vi "Menu_Case Selector Terminal.vi"(11 "Affected Items":T1) -> (3 "Menu Items To Add":T2(array[cluster]))   [LabVIEW 2023]
uses:
  top/BundleMagic.ctl
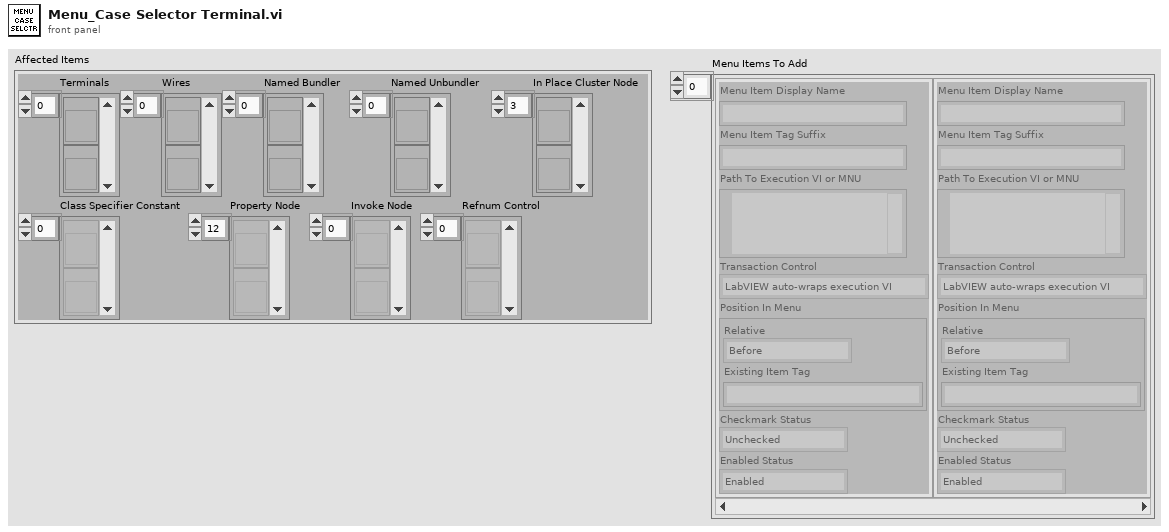
[diagram p1: front panel]
types:
  T1 = typedef "BundleMagic.ctl" = cluster{"Terminals":refnum<vi>[], "Wires":refnum<vi>[], "Named Bundler":refnum<vi>[], "Named Unbundler":refnum<vi>[], "In Place Cluster Node":refnum<vi>[], "Class Specifier Constant":refnum<vi>[], "Property Node":refnum<vi>[], "Invoke Node":refnum<vi>[], "Refnum Control":refnum<vi>[]}
  T2 = cluster{"Menu Item Display Name":string, "Menu Item Tag Suffix":string, "Path To Execution VI or MNU":path, "Transaction Control":enum8{"LabVIEW auto-wraps execution VI", "Execution VI will define if needed"}, "Position In Menu":cluster{"Relative":enum8{"Before", "Instead of", "After", "Into Submenu"}, "Existing Item Tag":string}, "Checkmark Status":enum8{"Unchecked", "Checked"}, "Enabled Status":enum8{"Enabled", "Disabled"}}[]
  T3 = cluster{"Relative":enum8{"Before", "Instead of", "After", "Into Submenu"}, "Existing Item Tag":string}
  T4 = enum16{"[NONE]", "Wire Bundle", "Wire Unbundle", "Terminal Unbundle", "Terminal Bundle", "Bundler Insert", "Bundler Remove", "Bundler Remove Unwired", "Bundler Rearrange", "In Place Insert", "In Place Remove", "In Place Remove Unwired", "In Place Rearrange", "Wire Properties", "Wire Method", "Terminal Properties", "Terminal Method", "Properties Insert", "Properties Remove", "Properties Remove Unwired", "Properties Rearrange", "Method Change", "Class for Constant", "Class For Control", "Class For Node", "Class Name to Clipboard"}[]
  T5 = cluster{"Relative":enum8{"Before", "Instead of", "After", "Into Submenu"}, "Existing Item Tag":string}[]
  T6 = cluster{"Menu Item Display Name":string, "Menu Item Tag Suffix":string, "Path To Execution VI or MNU":path, "Transaction Control":enum8{"LabVIEW auto-wraps execution VI", "Execution VI will define if needed"}, "Position In Menu":cluster{"Relative":enum8{"Before", "Instead of", "After", "Into Submenu"}, "Existing Item Tag":string}, "Checkmark Status":enum8{"Unchecked", "Checked"}, "Enabled Status":enum8{"Enabled", "Disabled"}}
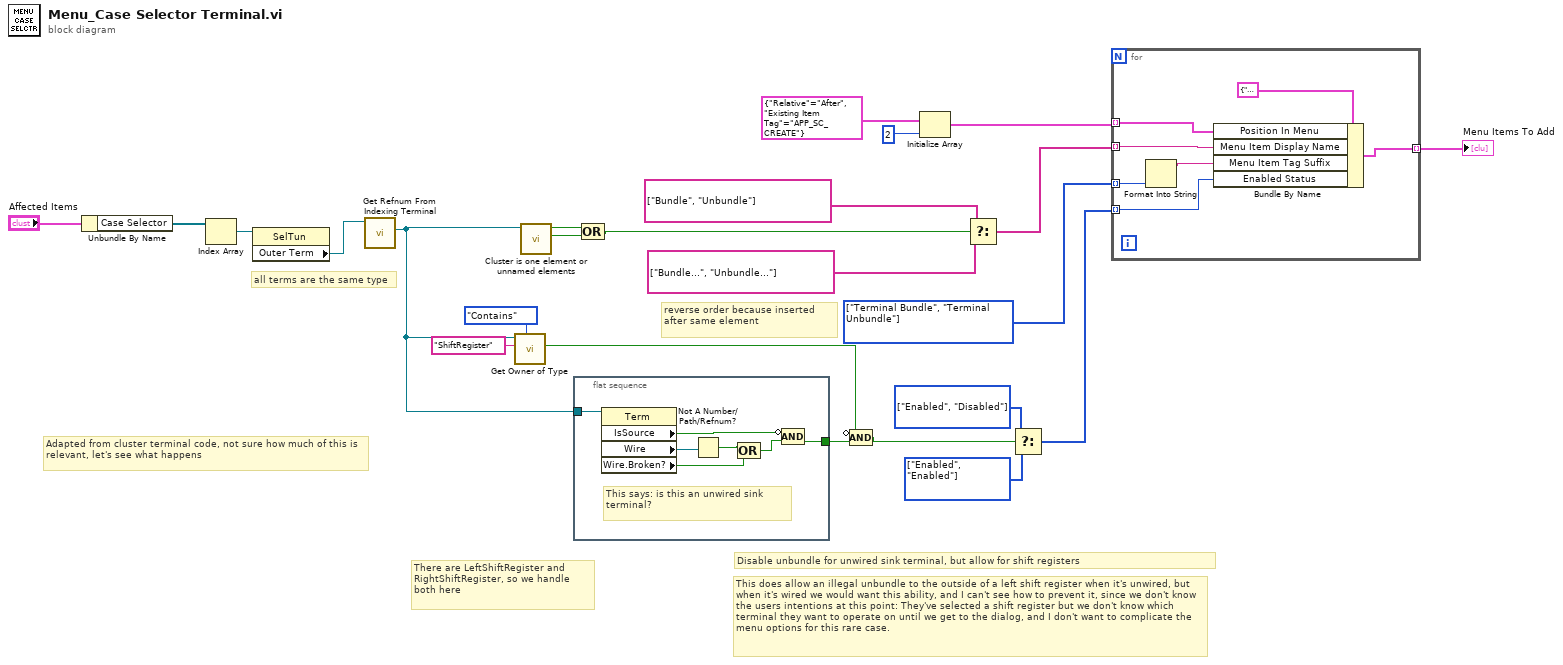
[diagram p0: block diagram]
diagram:
  w13 = T4 [enum."Terminal Bundle", enum."Terminal Unbundle"] items=["[NONE]", "Wire Bundle", "Wire Unbundle", "Terminal Unbundle", "Terminal Bundle", "Bundler Insert", "Bundler Remove", "Bundler Remove Unwired", "Bundler Rearrange", "In Place Insert", "In Place Remove", "In Place Remove Unwired", "In Place Rearrange", "Wire Properties", "Wire Method", "Terminal Properties", "Terminal Method", "Properties Insert", "Properties Remove", "Properties Remove Unwired", "Properties Rearrange", "Method Change", "Class for Constant", "Class For Control", "Class For Node", "Class Name to Clipboard"] ("Enabled Status")
  w21 = enum8{"Enabled", "Disabled"}[] [enum."Enabled", enum."Enabled"] items=["Enabled", "Disabled"] ("Enabled Status")
  w20 = enum8{"Enabled", "Disabled"}[] [enum."Enabled", enum."Disabled"] items=["Enabled", "Disabled"] ("Enabled Status")
  # "Adapted from cluster terminal code, not sure how much of this is relevant, let's see what happens"
  # "all terms are the same type"
  # "There are LeftShiftRegister and RightShiftRegister, so we handle both here"
  # "This does allow an illegal unbundle to the outside of a left shift register when it's unwired, but when it's wired we would want this ability, and I can't see how to prevent it, since we don't know the users intentions at this point: They've selected a shift register but we don't know which terminal they want to operate on until we get to the dialog, and I don't want to complicate the menu options for this rare case."
  # "reverse order because inserted after same element"
  # "Disable unbundle for unwired sink terminal, but allow for shift registers"
  n1 = Unbundle By Name("Affected Items") -> ("Case Selector"=w3:refnum<vi>[])
  n2 = Index Array(array=w3) -> (element=w2:refnum<vi>)  [unwired: 1 in]
  n3 = property class="SelTun"(reference=w2) -> ("Outer Term"=w1:refnum<vi>)  [unwired: 1 in, 2 out]
  n4 = call "Get Refnum From Indexing Terminal.vi"("Refnum Terminal"=w1) -> ("Chosen Terminal"=w6:refnum<vi>)  [unwired: 8 in, 2 out]
  n5 = call "Get Owner of Type.vi"("Match Type"=enum16{"Exact Match", "Contains"}."Contains", "Owner Class Name desired"="ShiftRegister", "reference"=w6) -> ("Owner of type found?"=w14:bool)  [unwired: 4 in, 4 out]
  n6 = call "Cluster is one element or unnamed elements.vi"("Cluster Terminal"=w6) -> ("All Unnamed?"=w8:bool, "One Element?"=w9:bool)  [unwired: 8 in, 1 out]
  n7 = flat-sequence {
    tunnel: [w27] -> w16
    tunnel: w6 -> [w26]
    frame #0 {
      # "This says: is this an unwired sink terminal?"
      n8 = property class="Term"(reference=w26) -> ("IsSource"=w25:bool, "Wire"=w31:refnum<vi>, "Wire.Broken?"=w29:bool)  [unwired: 1 in, 2 out]
      n9 = Not A Number/Path/Refnum?(number/path/refnum=w31) -> (NaN/Path/Refnum?=w30:bool)
      n10 = Compound Arithmetic op=OR(w30, w29) -> (w28:bool)
      n11 = Compound Arithmetic op=AND(invert w25, w28) -> (w27:bool)
    }
  }
  n12 = Compound Arithmetic op=OR(w9, w8) -> (w7:bool)
  n13 = Compound Arithmetic op=AND(invert w14, w16) -> (w15:bool)
  n14 = Initialize Array(T3 {"Relative"=enum."After", "Existing Item Tag"="APP_SC_CREATE"} ("Position In Menu"), 2) -> (w23:T5)
  n15 = Select(t=string[] ["Bundle", "Unbundle"], s=w7, f=string[] ["Bundle...", "Unbundle..."]) -> (s? t:f=w10:string[])
  n16 = Select(t=w20, s=w15, f=w21) -> (s? t:f=w19:enum8{"Enabled", "Disabled"}[])
  n17 = for {
    tunnel: [w36] -> w24 mode=indexing
    tunnel: w23 -> [w34] mode=indexing
    tunnel: w10 -> [w37] mode=indexing
    tunnel: w19 -> [w35] mode=indexing
    tunnel: w13 -> [w32] mode=indexing
    n18 = Format Into String(w32) -> (resulting string=w33:string)  [unwired: 3 in, 1 out]
    n19 = Bundle By Name(cluster=T6 {"Menu Item Display Name"="", "Menu Item Tag Suffix"="", "Path To Execution VI or MNU"=path "", "Transaction Control"=enum."LabVIEW auto-wraps execution VI", "Position In Menu"={"Relative"=enum."Before", "Existing Item Tag"=""}, "Checkmark Status"=enum."Unchecked", "Enabled Status"=enum."Enabled"} ("Cluster"), "Position In Menu"=w34, "Menu Item Display Name"=w37, "Menu Item Tag Suffix"=w33, "Enabled Status"=w35) -> (w36:T6)
  }
  "Menu Items To Add" <- w24
